vi "Toggle Relay.vi"(8 "error in":errorcluster, 9 "Relay State":bool, 10 "Relay Name":string, 11 "2525 in":refnum<class "2525.lvclass">) -> (0 "error out":errorcluster, 3 "2525 out":refnum<class "2525.lvclass">)   [LabVIEW 2019, in "2525.lvlib" / "2525.lvclass"]
doc: "Set one relay state to either on or off."
uses:
  Library/2525.lvclass
  Library/2525.lvclass/2525.ctl
  builds/Instruments/SwitchMatrix.lvlibp/Library/SwitchMatrix.lvclass
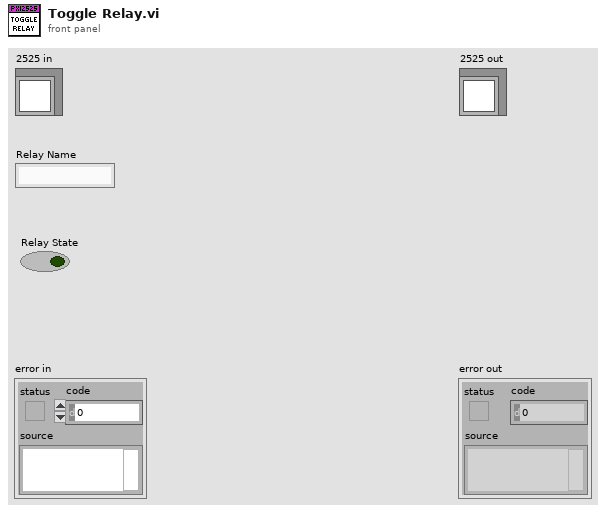
[diagram p1: front panel]
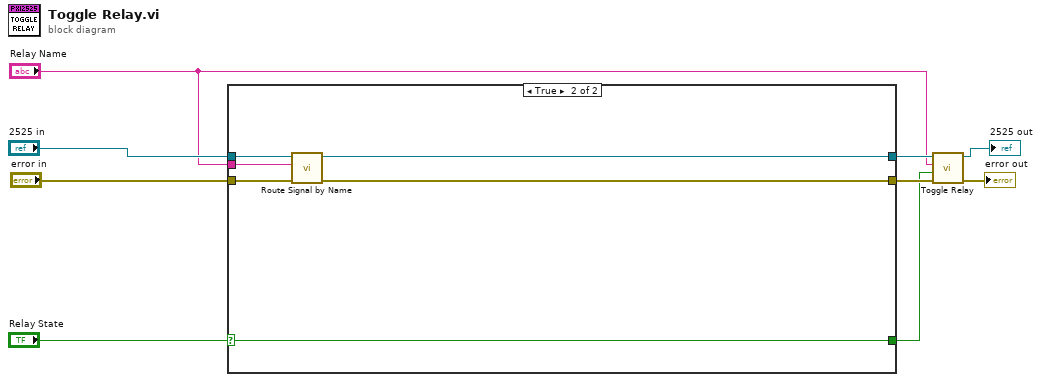
[diagram p0: block diagram]
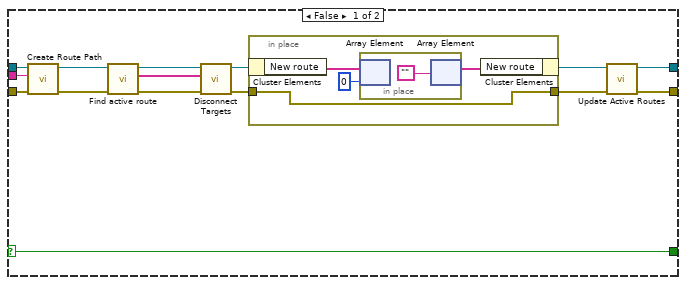
[diagram p2: hidden frame]
diagram:
  n1 = case shown="True" "Relay State" {
    selector: "Relay State" -> [w10 w30]
    tunnel: "2525 in" -> [w18 w35]
    tunnel: [w23 w34] -> w6
    tunnel: "Relay Name" -> [w17 w33]
    tunnel: "error in" -> [w16 w32]
    tunnel: [w24 w31] -> w5
    tunnel: [w10 w30] -> w1
    frame False {
      n2 = call "Create Route Path.vi"("error in"=w16, "Source"=w17, "2525 in"=w18) -> ("error out"=w15:errorcluster, "2525 out"=w14:refnum<class "2525.lvclass">)  [unwired: 7 in]
      n3 = call "Find active route.vi"("error in"=w15, "2525 in"=w14) -> ("error out"=w12:errorcluster, "Active Route"=w11:string[], "2525 out"=w13:refnum<class "2525.lvclass">)  [unwired: 7 in]
      n4 = call "Disconnect Targets.vi"("error in"=w12, "Disconnect targets"=w11, "2525 in"=w13) -> ("error out"=w20:errorcluster, "2525 out"=w22:refnum<class "2525.lvclass">)  [unwired: 7 in]
      n5 = in-place {
        in-place-border: w20 -> [w25]
        in-place-border: [w25] -> w19
        n6 = in-place-cluster #1(w22) -> ("New route"=w28:string[])
        n7 = in-place {
          n8 = in-place-array #2(w28, 0) -> ()  [unwired: 1 out]
          n9 = in-place-array #2("") -> (w27:string[])  [unwired: 1 out]
        }
        n10 = in-place-cluster #1("New route"=w27) -> (w21:refnum<class "2525.lvclass">)
      }
      n11 = call "Update Active Routes.vi"("error in"=w19, "2525 in"=w21) -> ("error out"=w24:errorcluster, "2525 out"=w23:refnum<class "2525.lvclass">)  [unwired: 8 in]
    }
    frame True {
      n12 = call-dynamic "Route Signal by Name.vi"("error in"=w32, "Source"=w33, "2525 in"=w35) -> ("error out"=w31:errorcluster, "2525 out"=w34:refnum<class "2525.lvclass">)  [unwired: 7 in]
    }
  }
  n13 = call-parent "Toggle Relay.vi"("error in"=w5, "Relay State"=w1, "Relay Name"="Relay Name", "SwitchMatrix in"=w6) -> ("error out"=→"error out":errorcluster, "SwitchMatrix out"=→"2525 out":refnum<class "2525.lvclass">)  [unwired: 6 in]
